vi "VK-1701Load Coating.vi"() -> (1 "Recipe":string[](array[string]), 2 "Coating Name":string, 3 "Path Array":string[](array[string]))   [LabVIEW 2009]
uses:
  <vilib>/Utility/file.llb/Read From Spreadsheet File (string).vi
panel:
  out "Experiment_path":path
  out "Cancelled":bool
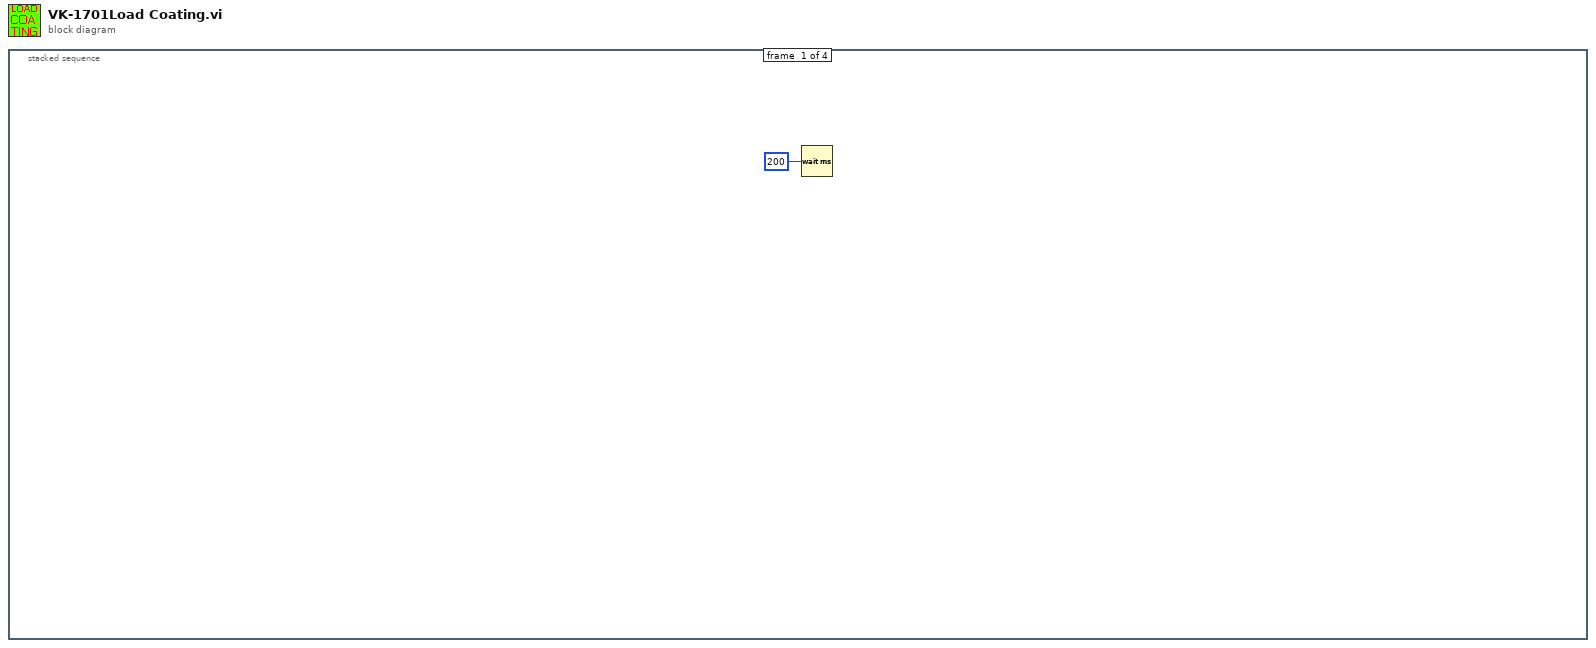
[diagram p0: block diagram]
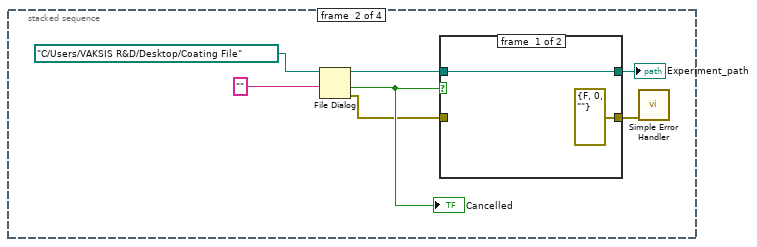
[diagram p2: hidden frame]
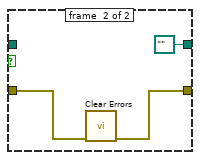
[diagram p3: hidden frame]
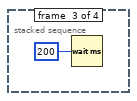
[diagram p4: hidden frame]
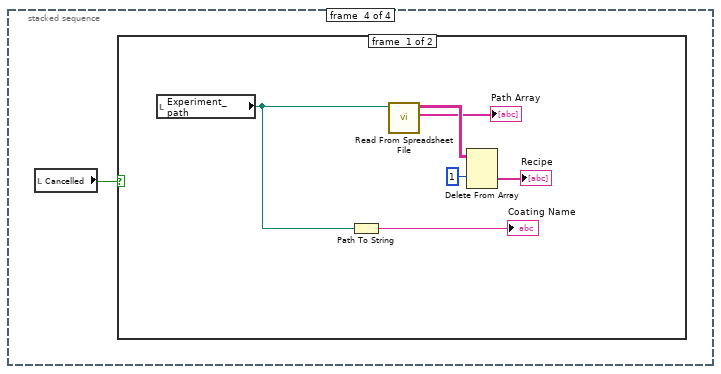
[diagram p5: hidden frame]
diagram:
  n1 = stacked-sequence {
    frame #0 {
      n2 = Wait (ms)(milliseconds to wait=u32 200) -> ()  [unwired: 1 out]
    }
    frame #1 {
      n3 = File Dialog(9:"" ("Path"), 11:path "C:/Users/VAKSIS R&D/Desktop/Coating File" ("base path")) -> (0:w5:errorcluster, 1:w6:bool, 3:w4:path)  [unwired: 2 in, 4 out]
      "Cancelled" <- w6
      n4 = case shown="False" w6 {
        tunnel: w5 -> [_ w13]
        tunnel: [w10 path ""] -> w2
        tunnel: w4 -> [w10 _]
        tunnel: [errorcluster {"status"=FALSE, "code"=0, "source"=""} ("error out") w12] -> w3
        frame #0 {
        }
        frame #1 {
          n5 = call <vilib>:"Clear Errors.vi"("error in (no error)"=w13) -> ("error out"=w12:errorcluster)  [unwired: 6 in]
        }
      }
      "Experiment_path" <- w2
      n6 = call <vilib>:"Simple Error Handler.vi"("error in (no error)"=w3) -> ()  [unwired: 4 in, 5 out]
    }
    frame #2 {
      n7 = Wait (ms)(milliseconds to wait=u32 200) -> ()  [unwired: 1 out]
    }
    frame #3 {
      n8 = local read "Cancelled"() -> (w15:bool)
      n9 = case shown="False" w15 {
        frame #0 {
          n10 = local read "Experiment_path"() -> (w16:path)
          n11 = Path To String(path=w16) -> (string=→"Coating Name":string)
          n12 = call-poly <vilib>:"Read From Spreadsheet File.vi"("file path (dialog if empty)"=w16) -> ("first row"=→"Path Array":string[], "all rows"=w20:string[][])  [unwired: 6 in, 3 out]
          n13 = Delete From Array(array=w20, index (row)=1) -> (deleted portion=→"Recipe":string[])  [unwired: 2 in, 1 out]
        }
        frame #1 {
        }
      }
    }
  }
